vi "FTW-Actor-Core-SpawnHandshake.vi"(0 "Actor Spawn Options":T2={"HandshakeTimeout"=2000, "Handshaker"=refnum, "ShowPanelSpecified"=TRUE, "ShowPanelValue"=TRUE} {"HandshakeTimeout" format="%d msec"}, 11 "error in":errorcluster) -> (4 "FTW Actor Connector":T1, 6 "Instance Inbox Address":string, 8 "Instance VI Clone Name":string, 15 "error out":errorcluster)   [LabVIEW 2015]
uses:
  FTW-Actor-Core-SpawnOptions.ctl
  core/type/FTW-Type-JSON.ctl
  core/type/FTW-Type-Actor-Connector.ctl
  json/core/FTW-JSON-Core-Type.ctl
  reflection/FTW-Reflection-Types.ctl
  lib/FTW-KernelFilepath.vi
  codegen/xnode/json/fetch/FTW-JSON-Core-GetFlattenedValue.vi
  json/core/FTW-JSON-Core-LibraryReturnValue.vi
  error/FTW-ERR-ThrowInvalidReferenceError.vi
  json/core/FTW-JSON-Core-ElementType.vi
  codegen/xnode/FTW-JSON-Fetch.xnode
  json/FTW-JSON-Type.ctl
panel:
  # "Inputs"
  # "Outputs"
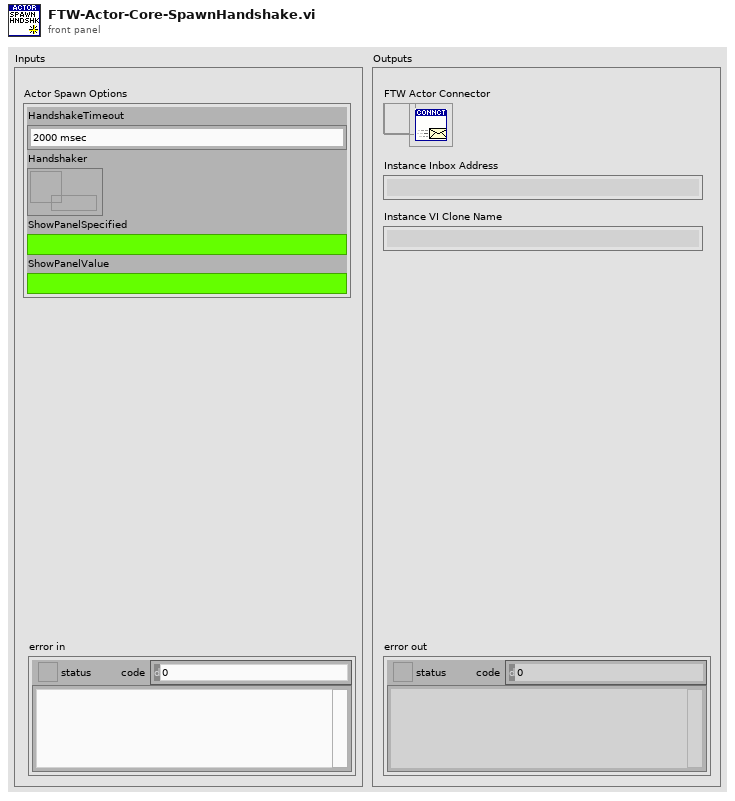
[diagram p1: front panel]
types:
  T1 = typedef "FTW-Type-Actor-Connector.ctl" = refnum<data-value>
  T2 = typedef "FTW-Actor-Core-SpawnOptions.ctl" = cluster{"HandshakeTimeout":i32, "Handshaker":refnum<queue>, "ShowPanelSpecified":bool, "ShowPanelValue":bool}
  T3 = cluster{"FTW-PrimaryInboxAddress":string, "FTW-InstanceCloneName":string}
  T4 = typedef "FTW-JSON-Core-Type.ctl" = enum8{"Object", "Array", "String", "Integer", "Floating Point", "true", "false", "null", "undefined"}
  T5 = typedef "FTW-Type-JSON.ctl" = refnum<data-value>
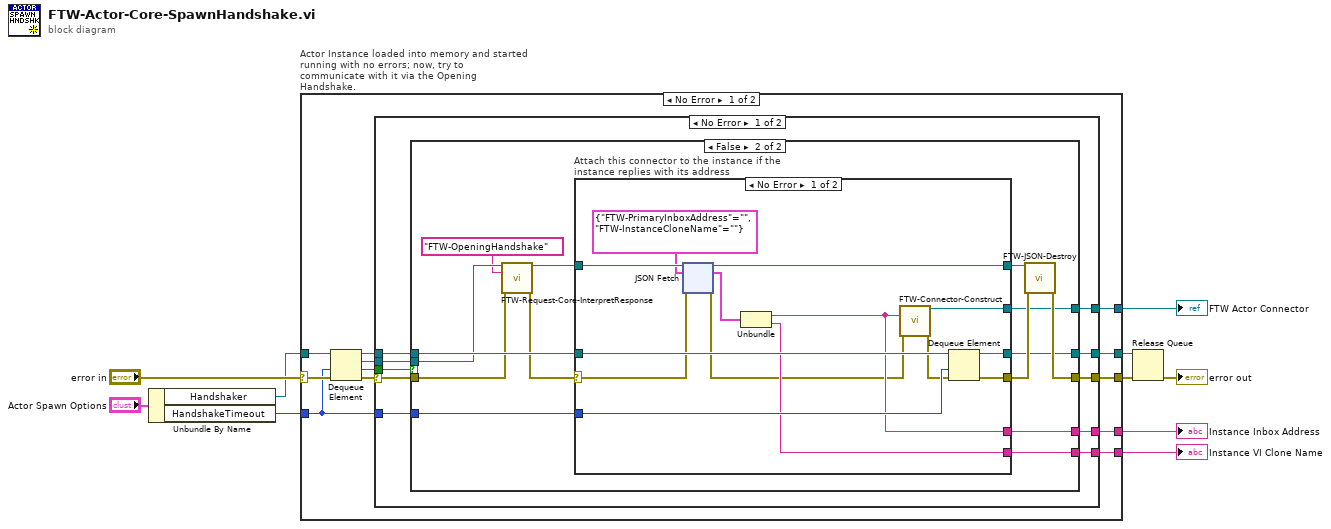
[diagram p0: block diagram]
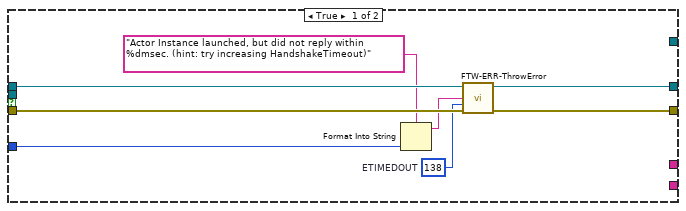
[diagram p2: hidden frame]
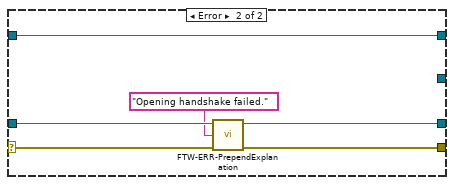
[diagram p3: hidden frame]
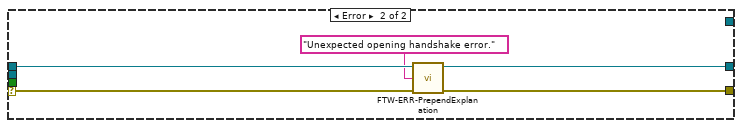
[diagram p4: hidden frame]
diagram:
  n1 = Unbundle By Name("Actor Spawn Options") -> ("Handshaker"=w4:refnum<queue>, "HandshakeTimeout"=w3:i32)
  n2 = case "Actor Instance loaded into memory and started running with no errors; now, try to communicate with it via the Opening Handshake." shown="No Error" "error in" {
    selector: "error in" -> [w17 w131]
    tunnel: [w22 w131] -> w9
    tunnel: [w21 _] -> w1
    tunnel: w4 -> [w19 w130]
    tunnel: [w20 w130] -> w10
    tunnel: w3 -> [w15 _]
    tunnel: [w12 _] -> w7
    tunnel: [w11 _] -> w6
    frame No Error {
      n3 = Dequeue Element(queue=w19, timeout in ms (-1)=w15, error in (no error)=w17) -> (queue out=w18:refnum<queue>, element=w16:T5, timed out?=w14:bool, error out=w13:errorcluster)
      n4 = case shown="No Error" w13 {
        selector: w13 -> [w25 w128]
        tunnel: [w32 w127] -> w22
        tunnel: [w31 _] -> w21
        tunnel: [w30 w129] -> w20
        tunnel: w18 -> [w29 w129]
        tunnel: w16 -> [w28 _]
        tunnel: w15 -> [w27 _]
        tunnel: w14 -> [w26 _]
        tunnel: [w24 _] -> w12
        tunnel: [w23 _] -> w11
        frame No Error {
          n5 = case shown="False" w26 {
            tunnel: [w34 w45] -> w32
            tunnel: [_ w41] -> w31
            tunnel: w29 -> [w38 w53]
            tunnel: [w38 w40] -> w30
            tunnel: w27 -> [w36 w52]
            tunnel: w28 -> [_ w48]
            tunnel: w25 -> [w39 w49]
            tunnel: [_ w51] -> w24
            tunnel: [_ w50] -> w23
            frame True {
              w35 = 138  # ETIMEDOUT
              n6 = Format Into String(format string="Actor Instance launched, but did not reply within %dmsec. (hint: try increasing HandshakeTimeout)" ("Error Message"), w36) -> (resulting string=w33:string)  [unwired: 2 in, 1 out]
              n7 = call "FTW-ERR-ThrowError.vi"("Error Message"=w33, "Error Code"=w35, "error in"=w39) -> ("error out"=w34:errorcluster)  [unwired: 12 in]
            }
            frame False {
              n8 = call "FTW-Request-Core-InterpretResponse.vi"("Raw Response"=w48, "Expected Request Header"="FTW-OpeningHandshake" ("Request Header"), "error in"=w49) -> ("InterpretedResponse"=w47:T5, "error out"=w43:errorcluster)  [unwired: 11 in]
              n9 = case "Attach this connector to the instance if the instance replies with its address" shown="No Error" w43 {
                selector: w43 -> [w55 w123]
                tunnel: [w66 _] -> w41
                tunnel: [w64 w125] -> w44
                tunnel: w53 -> [w67 w124]
                tunnel: [w65 w124] -> w40
                tunnel: w52 -> [w63 _]
                tunnel: [w57 _] -> w51
                tunnel: [w56 _] -> w50
                tunnel: w47 -> [w61 w121]
                tunnel: [w60 w121] -> w46
                frame No Error {
                  n10 = xnode "JSON Fetch"("JSON"=w61, "Element Type and Default Value"=T3 {"FTW-PrimaryInboxAddress"="", "FTW-InstanceCloneName"=""}, "error in"=w55) -> ("JSON out"=w60:T5, "Value"=w58:T3, "error out"=w54:errorcluster)  [unwired: 2 in, 1 out]
                  n11 = Unbundle(w58) -> ("FTW-PrimaryInboxAddress"=w57:string, "FTW-InstanceCloneName"=w56:string)
                  n12 = call "FTW-Connector-Construct.vi"("Remote Inbox Address"=w57, "error in"=w54) -> ("Actor Connector"=w66:T1, "error out"=w62:errorcluster)  [unwired: 12 in]
                  n13 = Dequeue Element(queue=w67, timeout in ms (-1)=w63, error in (no error)=w62) -> (queue out=w65:refnum<queue>, error out=w64:errorcluster)  [unwired: 2 out]
                }
                frame Error {
                  n14 = call "FTW-ERR-PrependExplanation.vi"("Exception Information"="Opening handshake failed.", "error in"=w123) -> ("error out"=w125:errorcluster)  [unwired: 13 in]
                }
              }
              n15 = call "FTW-JSON-Destroy.vi"("JSON"=w46, "error in"=w44) -> ("error out"=w45:errorcluster)  [unwired: 13 in]
            }
          }
        }
        frame Error {
          n16 = call "FTW-ERR-PrependExplanation.vi"("Exception Information"="Unexpected opening handshake error.", "error in"=w128) -> ("error out"=w127:errorcluster)  [unwired: 13 in]
        }
      }
    }
    frame Error {
    }
  }
  "Instance Inbox Address" <- w7
  "Instance VI Clone Name" <- w6
  "FTW Actor Connector" <- w1
  n17 = Release Queue(queue=w10, error in (no error)=w9) -> (error out=→"error out":errorcluster)  [unwired: 1 in, 2 out]
